vi "mupDefineVar_Array.vi"(8 "error in (no error)":errorcluster, 9 "initValue":dbl[](array[numeric]), 10 "varName":string, 11 "hParser in":u64) -> (0 "error out":errorcluster, 2 "varAddr":u64, 3 "hParser out":u64)   [LabVIEW 2015, in "mupLib.lvlib"]
doc: "Define a variable and set its initial values for bulk mode evaluation.\nThe variable's pointer is returned in varAddr."
uses:
  mupLib.lvlib
  <vilib>/Utility/error.llb/Error Cluster From Error Code.vi
panel:
  # "Define a variable and set its initial values for bulk mode evaluation.\nThe variable's pointer is returned in varAddr."
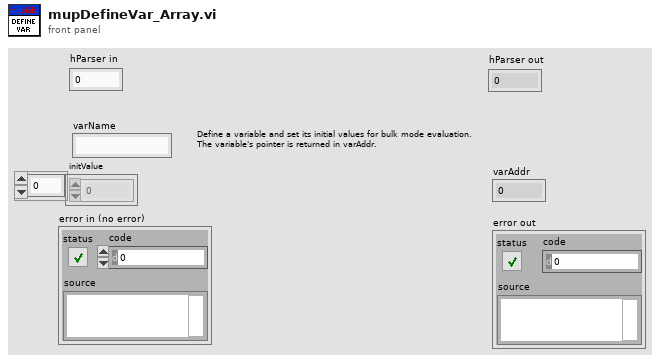
[diagram p1: front panel]
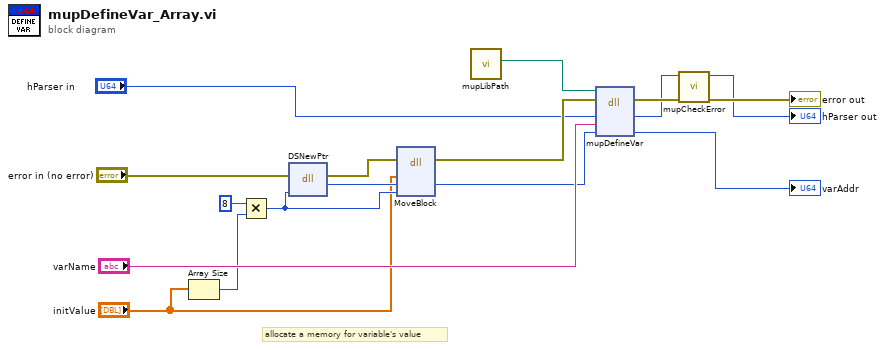
[diagram p0: block diagram]
diagram:
  # "allocate a memory for variable's value"
  n1 = Array Size(array="initValue") -> (size(s)=w1:i32)
  n2 = Multiply(x=8 ("size"), y=w1) -> (x*y=w3:i32)
  n3 = dll-call lib="LabVIEW" fn="DSNewPtr"(error in="error in (no error)", "size"=w3) -> (error out=w16:errorcluster, "return type"=w17:u64)  [unwired: 3 in, 1 out]
  n4 = dll-call lib="LabVIEW" fn="MoveBlock"(error in=w16, "ps"="initValue", "pd"=w17, "size"=w3) -> (error out=w15:errorcluster, "pd"=w13:u64)  [unwired: 5 in, 1 out]
  n5 = call "mupLibPath.vi"() -> ("libmuparser path"=w5:path)  [unwired: 11 in]
  n6 = dll-call lib="usr/lib/x86_64-linux-gnu/libmuparser.so.2" fn="mupDefineVar"(path in=w5, error in=w15, "hParser"="hParser in", "szName"="varName", "fVar"=w13) -> (error out=w10:errorcluster, "hParser"=w6:u64, "fVar"=→"varAddr":u64)  [unwired: 3 in, 1 out]
  n7 = call "mupCheckError.vi"("error in (no error)"=w10, "hParser in"=w6) -> ("error out"=→"error out":errorcluster, "hParser out"=→"hParser out":u64)  [unwired: 8 in]
